vi "loadMessages.vi"(8 "error in (no error)":errorcluster, 9 "FileName (without extension)":string="messages", 10 "TextDisplay":refnum<class "TextDisplay Class.lvclass">) -> (0 "error out":errorcluster, 3 "simonMessages out":refnum<class "simonMessages.lvclass">)   [LabVIEW 2020, in "simonMessages.lvclass"]
uses:
  simonMessages.lvclass
  TextDisplay/TextDisplay Class.lvclass
  simonMessages.lvclass/simonMessages.ctl
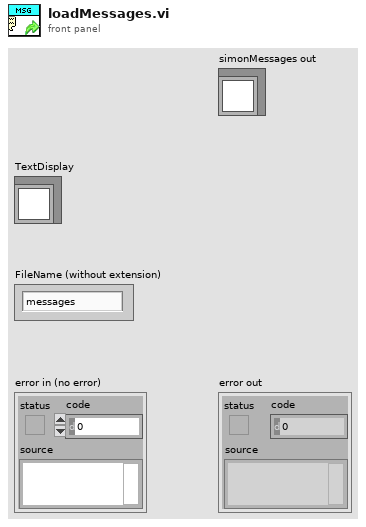
[diagram p1: front panel]
types:
  T1 = enum16{"open", "replace", "create", "open or create", "replace or create", "replace or create with confirmation"}
  T2 = map{string, cluster{"Text":string, "Size":u8, "Justification":enum16{"Left", "Center", "Right"}, "Display Type":string}}
  T3 = map{string, cluster{"Text":string, "Size":u8, "Justification":enum16{"Left", "Center", "Right"}, "Display Type":string}}[]
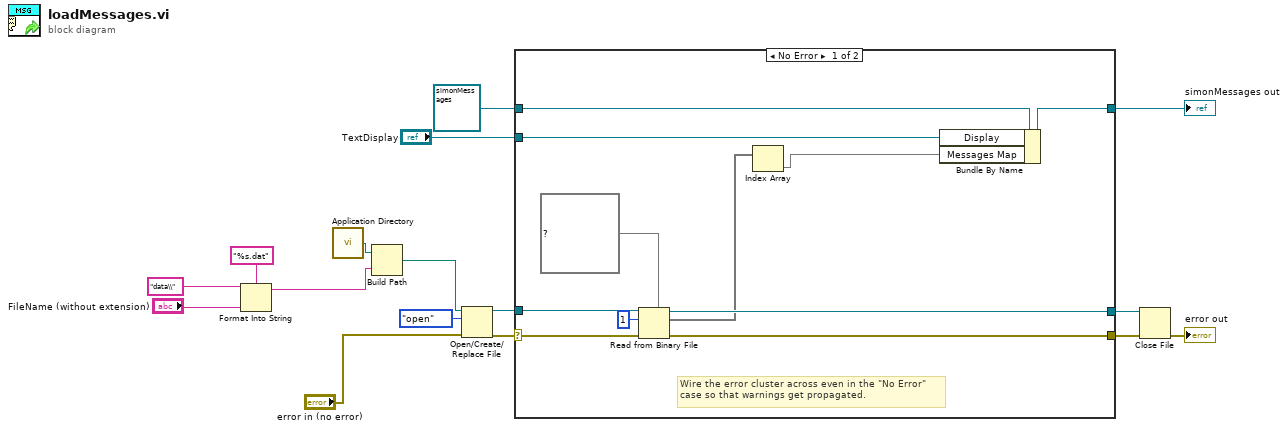
[diagram p0: block diagram]
diagram:
  n1 = Format Into String(format string="%s.dat" ("name or relative path"), initial string="data\\" ("name or relative path"), "FileName (without extension)") -> (resulting string=w4:string)  [unwired: 1 in, 1 out]
  n2 = call <vilib>:"Application Directory.vi"() -> ("Application Directory"=w6:path)
  n3 = Build Path(base path=w6, name or relative path=w4) -> (appended path=w2:path)
  n4 = Open/Create/Replace File(file path (use dialog)=w2, error in="error in (no error)", operation (0:open)=T1."open") -> (refnum out=w11:refnum<file>, error out=w10:errorcluster)  [unwired: 3 in, 1 out]
  n5 = case shown="No Error" w10 {
    selector: w10 -> [w26 w30]
    tunnel: [w25 w30] -> w16
    tunnel: [w21 w29] -> w14
    tunnel: refnum<class "simonMessages.lvclass"> refnum ("simonMessages in") -> [w27 w29]
    tunnel: w11 -> [w24 w28]
    tunnel: [w23 w28] -> w8
    tunnel: "TextDisplay" -> [w20 _]
    frame No Error {
      # "Wire the error cluster across even in the \"No Error\"\ncase so that warnings get propagated."
      n6 = Read from Binary File(5:T2 {} ("Messages Map"), 8:w26, 10:1 ("count (1)"), 11:w24) -> (0:w25:errorcluster, 2:w19:T3, 3:w23:refnum<file>)  [unwired: 2 in, 1 out]
      n7 = Index Array(array=w19) -> (element=w17:T2)  [unwired: 1 in]
      n8 = Bundle By Name(cluster=w27, "Display"=w20, "Messages Map"=w17) -> (w21:refnum<class "simonMessages.lvclass">)
    }
    frame Error {
    }
  }
  "simonMessages out" <- w14
  n9 = Close File(refnum=w8, error in=w16) -> (error out=→"error out":errorcluster)  [unwired: 1 out]
